vi "polymorphic GFGpolyGet - Example.vi"() -> ()   [LabVIEW 2012]
doc: "SciScan 1.2 160622"
uses:
  <vilib>/Utility/miscctls.llb/LVMinMaxIncTypeDef.ctl
  GFGbooleanGet.vi
  GFGnumericGet.vi
  GFGstringGet.vi
  GFGpathGet.vi
  GFGfpRefGet.vi
  GFGImageRefsGet.vi
  GFG library.lvlib
panel:
  out "Data Entry Limits":T1
  out "Channel 1 large":T2(plugin-control)
  out "Path":path
  out "String":string
  out "Numeric":dbl
  out "Boolean":bool
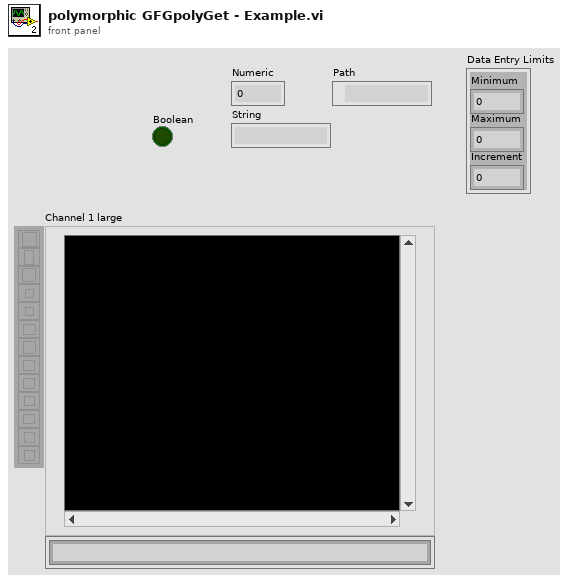
[diagram p1: front panel]
types:
  T1 = typedef "LVMinMaxIncTypeDef.ctl" = cluster{"Minimum":dbl, "Maximum":dbl, "Increment":dbl}
  T2 = typedef "IMAQ Image.ctl" = refnum<image>
  T3 = cluster{"WaveformChartRef":refnum<vi>, "DigitalRef":refnum<vi>, "ArrayRef":refnum<vi>, "TabControlRef":refnum<vi>, "EnumRef":refnum<vi>, "RingRef":refnum<vi>, "BooleanRef":refnum<vi>, "KnobRef":refnum<vi>, "SlideRef":refnum<vi>, "PathRef":refnum<vi>, "StringRef":refnum<vi>, "ComboBox":refnum<vi>, "WaveformGraphRef":refnum<vi>}
  T4 = cluster{"Channel 1 small":T2, "Channel 2 small":T2, "Channel 3 small":T2, "Channel 4 small":T2, "Channel 1 large":T2, "Channel 2 large":T2, "Channel 3 large":T2, "Channel 4 large":T2, "RGB overlay":T2, "ROI Image display":T2, "arb line scan display":T2, "Channel 5 large":T2}
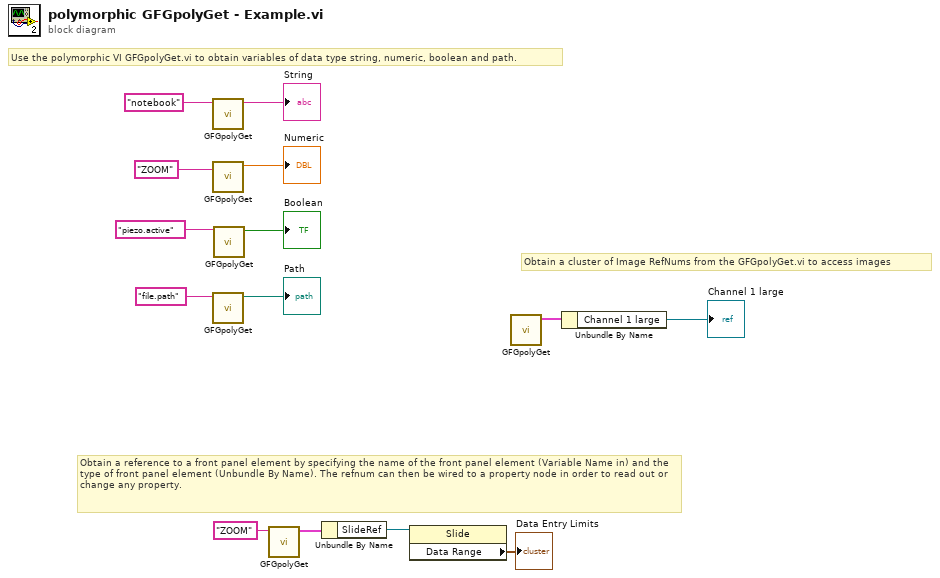
[diagram p0: block diagram]
diagram:
  # "Obtain a reference to a front panel element by specifying the name of the front panel element (Variable Name in) and the type of front panel element (Unbundle By Name). The refnum can then be wired to a property node in order to read out or change any property."
  # "Obtain a cluster of Image RefNums from the GFGpolyGet.vi to access images"
  # "Use the polymorphic VI GFGpolyGet.vi to obtain variables of data type string, numeric, boolean and path."
  n1 = call-poly "GFGpolyGet.vi"("Variable Name in"="notebook") -> ("String"=→"String":string)  [unwired: 9 in, 1 out]
  n2 = call-poly "GFGpolyGet.vi"("Variable Name in"="ZOOM") -> ("Numeric"=→"Numeric":dbl)  [unwired: 8 in, 2 out]
  n3 = call-poly "GFGpolyGet.vi"("Variable Name in"="file.path") -> ("Path"=→"Path":path)  [unwired: 8 in, 2 out]
  n4 = call-poly "GFGpolyGet.vi"("Variable Name in"="piezo.active") -> ("Boolean Value OUT"=→"Boolean":bool)  [unwired: 9 in, 1 out]
  n5 = call-poly "GFGpolyGet.vi"("Variable Name in"="ZOOM") -> ("output cluster"=w4:T3)  [unwired: 9 in, 1 out]
  n6 = Unbundle By Name(w4) -> ("SlideRef"=w2:refnum<vi>)
  n7 = property class="Slide"(reference=w2) -> ("Data Range"=→"Data Entry Limits":T1)  [unwired: 1 in, 2 out]
  n8 = call-poly "GFGpolyGet.vi"() -> ("Image Refs Out"=w6:T4)  [unwired: 10 in, 1 out]
  n9 = Unbundle By Name(w6) -> ("Channel 1 large"=→"Channel 1 large":T2)
